vi "sub_undoInvalidGuess.vi"(11 "queues":T1) -> ()   [LabVIEW 2018]
uses:
  guess.ctl
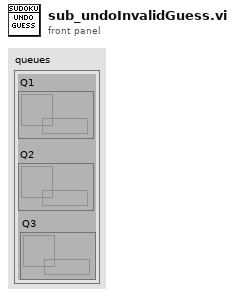
[diagram p1: front panel]
types:
  T1 = cluster{"Q1":refnum<queue>, "Q2":refnum<queue>, "Q3":refnum<queue>}
  T2 = typedef "guess.ctl" = cluster{"cell position":cluster{"row":i32, "col":i32}, "guess":string}
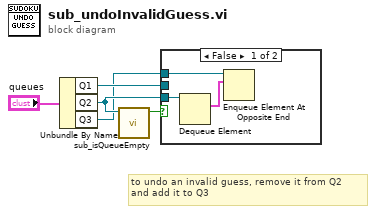
[diagram p0: block diagram]
diagram:
  # "to undo an invalid guess, remove it from Q2 \nand add it to Q3"
  n1 = Unbundle By Name("queues") -> ("Q1"=w4:refnum<queue>, "Q2"=w3:refnum<queue>, "Q3"=w2:refnum<queue>)
  n2 = call "sub_isQueueEmpty"("Q1"=w3) -> ("empty ?"=w5:bool)  [unwired: 10 in]
  n3 = case shown="False" w5 {
    tunnel: w4 -> [_ _]
    tunnel: w3 -> [w8 _]
    tunnel: w2 -> [w7 _]
    frame False {
      n4 = Dequeue Element(queue=w8) -> (element=w6:T2)  [unwired: 2 in, 3 out]
      n5 = Enqueue Element At Opposite End(queue=w7, element=w6) -> ()  [unwired: 2 in, 3 out]
    }
    frame True {
    }
  }
